vi "timeout.vi"(2 "vars in":T1={"wait count t"=0, "wait min"=0, "wait max"=0, "stim count t"=0, "stim count n"=0, "d stim"=0, "d timeout"=0, "timeout win"=0, "base temp"=0.0, "stim amps"=[], "n hit"=0, "n catch"=0, "active"=TRUE, "catch"=TRUE, "stimulus"=TRUE, "reward given"=TRUE, "pairing"=TRUE, "lick"=FALSE, "next reward"=FALSE, "clean tubes"=FALSE, "next temp"=0.0}) -> (7 "vars out":T1={"wait count t"=0, "wait min"=0, "wait max"=0, "stim count t"=0, "stim count n"=0, "d stim"=0, "d timeout"=0, "timeout win"=0, "base temp"=0.0, "stim amps"=[], "n hit"=0, "n catch"=0, "active"=TRUE, "catch"=TRUE, "stimulus"=TRUE, "reward given"=TRUE, "pairing"=TRUE, "lick"=FALSE, "next reward"=FALSE, "clean tubes"=FALSE, "next temp"=0.0})   [LabVIEW 2015]
uses:
  Type Definitions/vars.ctl
panel:
  # "(see Block Diagram)"
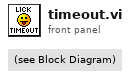
[diagram p1: front panel]
types:
  T1 = typedef "vars.ctl" = cluster{"wait count t":u16, "wait min":u16, "wait max":u16, "stim count t":u16, "stim count n":u16, "d stim":u16, "d timeout":u16, "timeout win":u16, "base temp":sgl, "stim amps":i32[], "n hit":u16, "n catch":u16, "active":bool, "catch":bool, "stimulus":bool, "reward given":bool, "pairing":bool, "lick":bool, "next reward":bool, "clean tubes":bool, "next temp":sgl}
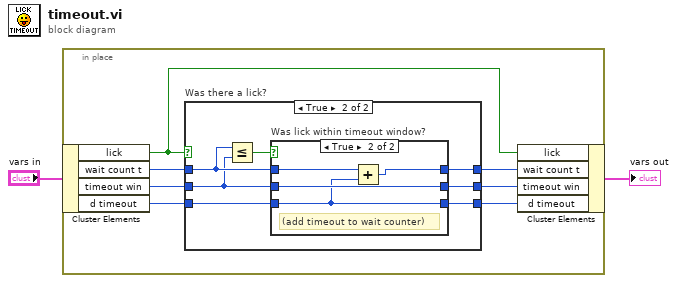
[diagram p0: block diagram]
diagram:
  n1 = in-place {
    n2 = in-place-cluster #1("vars in") -> ("lick"=w3:bool, "wait count t"=w9:u16, "timeout win"=w8:u16, "d timeout"=w7:u16)
    n3 = case "Was there a lick?" shown="True" w3 {
      tunnel: w9 -> [w12 w17]
      tunnel: w8 -> [w11 w15]
      tunnel: w7 -> [w10 w13]
      tunnel: [w12 w18] -> w6
      tunnel: [w11 w16] -> w5
      tunnel: [w10 w14] -> w4
      frame False {
        # "(do nothing)"
      }
      frame True {
        n4 = Less Or Equal?(x=w17, y=w15) -> (x <= y?=w19:bool)
        n5 = case "Was lick within timeout window?" shown="True" w19 {
          tunnel: [w22 w25] -> w18
          tunnel: w17 -> [w22 w23]
          tunnel: [w21 w26] -> w16
          tunnel: w15 -> [w21 w26]
          tunnel: [w20 w24] -> w14
          tunnel: w13 -> [w20 w24]
          frame False {
            # "(do nothing)"
          }
          frame True {
            # "(add timeout to wait counter)"
            n6 = Add(x=w23, y=w24) -> (x+y=w25:u16)
          }
        }
      }
    }
    n7 = in-place-cluster #1("lick"=w3, "wait count t"=w6, "timeout win"=w5, "d timeout"=w4) -> (→"vars out":T1)
  }
